vi "get sensor data.vi"() -> (0 "Ramp Belts Light Sensor":bool, 3 "Arm Actuator Limit Switches":cluster{"Boolean":bool, "Boolean":bool}, 4 "Shooter Cage Light Sensor":bool)   [LabVIEW 2015]
uses:
  <vilib>/Rock Robotics/Network Tables/NT Read Boolean.vi
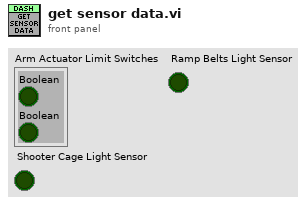
[diagram p1: front panel]
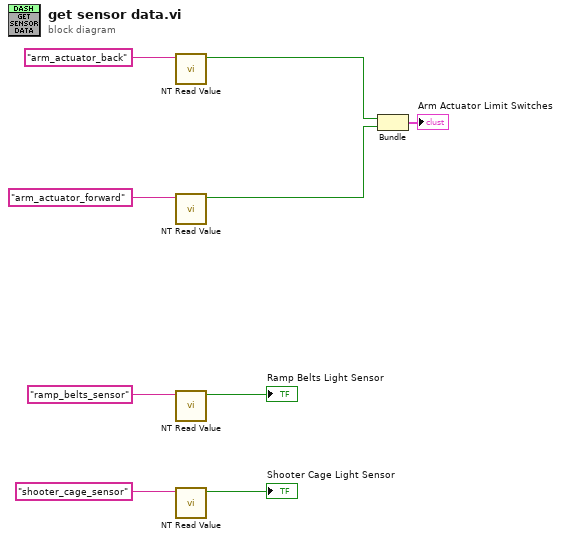
[diagram p0: block diagram]
diagram:
  n1 = call-poly <vilib>:"NT Read Value.vi"("Name"="arm_actuator_back") -> ("Boolean"=w6:bool)  [unwired: 9 in, 1 out]
  n2 = call-poly <vilib>:"NT Read Value.vi"("Name"="arm_actuator_forward") -> ("Boolean"=w4:bool)  [unwired: 9 in, 1 out]
  n3 = call-poly <vilib>:"NT Read Value.vi"("Name"="ramp_belts_sensor") -> ("Boolean"=→"Ramp Belts Light Sensor":bool)  [unwired: 9 in, 1 out]
  n4 = call-poly <vilib>:"NT Read Value.vi"("Name"="shooter_cage_sensor") -> ("Boolean"=→"Shooter Cage Light Sensor":bool)  [unwired: 9 in, 1 out]
  n5 = Bundle("Boolean"=w6, "Boolean"=w4) -> (→"Arm Actuator Limit Switches":cluster{"Boolean":bool, "Boolean":bool})  [unwired: 1 in]
